vi "McsaInitialize.vi"(8 "error in (no error)":errorcluster) -> (0 "error out":errorcluster, 3 "Qbus out":refnum<class "Qbus.lvclass">)   [LabVIEW 2017]
uses:
  <vilib>/addons/Qbus/Qbus.lvclass
  <vilib>/addons/TraceLogger/TraceLogger.lvlib
  <vilib>/addons/SystemInfoProcess/SystemInfoProcess.lvlib
  <vilib>/addons/InsightCM/Utilities/GlobalConfiguration/GlobalConfiguration.lvlib
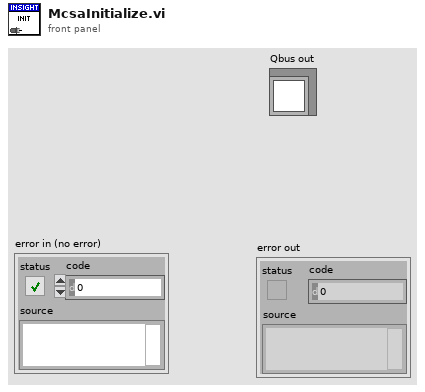
[diagram p1: front panel]
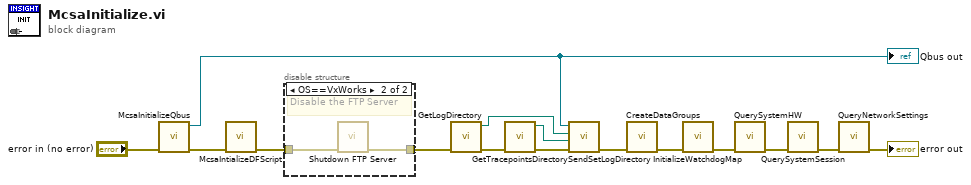
[diagram p0: block diagram]
diagram:
  n1 = call <vilib>:"McsaInitializeQbus.vi"("error in (no error)"="error in (no error)") -> ("error out"=w12:errorcluster, "Qbus out"=w13:refnum<class "Qbus.lvclass">)  [unwired: 9 in]
  "Qbus out" <- w13
  n2 = call <vilib>:"McsaIntializeDFScript.vi"("error in (no error)"=w12) -> ("error out"=w11:errorcluster)  [unwired: 10 in]
  n3 = disable-structure shown="OS==VxWorks" {
    disable-tunnel: [w16 w18] -> w7
    disable-tunnel: w11 -> [w16 w17]
    frame condition #0 (active) {
    }
    frame condition #1 {
      # "Disable the FTP Server"
      n4 = call <vilib>:"Shutdown FTP Server.vi"("error in (no error)"=w17) -> ("error out"=w18:errorcluster)  [unwired: 10 in]
    }
  }
  n5 = call <vilib>:"GetLogDirectory.vi"("error in (no error)"=w7) -> ("error out"=w3:errorcluster, "log dir"=w6:path)  [unwired: 9 in]
  n6 = call <vilib>:"GetTracepointsDirectory.vi"("error in (no error)"=w3) -> ("error out"=w1:errorcluster, "application directory"=w2:path)  [unwired: 9 in]
  n7 = call <vilib>:"SendSetLogDirectory.vi"("error in (no error)"=w1, "tracpoint directory"=w2, "log directory"=w6, "qbus in"=w13) -> ("error out"=w14:errorcluster)  [unwired: 6 in, 1 out]
  n8 = call <vilib>:"CreateDataGroups.vi"("error in (no error)"=w14) -> ("error out"=w5:errorcluster)  [unwired: 10 in]
  n9 = call <vilib>:"InitializeWatchdogMap.vi"("error in (no error)"=w5) -> ("error out"=w4:errorcluster)  [unwired: 10 in]
  n10 = call <vilib>:"QuerySystemHW.vi"("error in (no error)"=w4) -> ("error out"=w10:errorcluster)  [unwired: 10 in]
  n11 = call <vilib>:"QuerySystemSession.vi"("error in (no error)"=w10) -> ("error out"=w9:errorcluster)  [unwired: 10 in]
  n12 = call <vilib>:"QueryNetworkSettings.vi"("error in (no error)"=w9) -> ("error out"=→"error out":errorcluster)  [unwired: 10 in]
